vi "Write Delay.vi"(10 "Delay":u32 caption="Delay between writes (ms)", 11 "PIC-Device in":refnum<class "PIC-Device.lvclass">) -> (3 "PIC-Device out":refnum<class "PIC-Device.lvclass">)   [LabVIEW 2020, in "PIC-Device.lvclass"]
uses:
  PIC-Device.lvclass
  PIC-Device.lvclass/PIC-Device.ctl
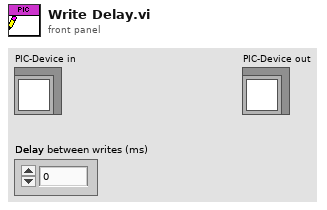
[diagram p1: front panel]
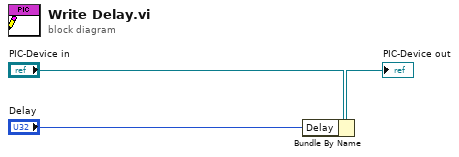
[diagram p0: block diagram]
diagram:
  n1 = Bundle By Name(cluster="PIC-Device in", "Delay"="Delay") -> (→"PIC-Device out":refnum<class "PIC-Device.lvclass">)
